vi "Setup Statically-Linked subWorkers.vi"(8 "error in":errorcluster, 11 "UI SmarAct in":refnum<class "UI SmarAct.lvclass">) -> (0 "error out":errorcluster, 3 "UI SmarAct out":refnum<class "UI SmarAct.lvclass">)   [LabVIEW 2024, in "UI SmarAct.lvclass"]
doc: "This VI performs a setup of all the statically-linked subWorkers that belong to the Worker that owns this VI. This VI must be called <b>before</b> any statically-linked subWorkers are called."
uses:
  UI SmarAct.lvclass
  UI SmarAct.lvclass/UI SmarAct.ctl
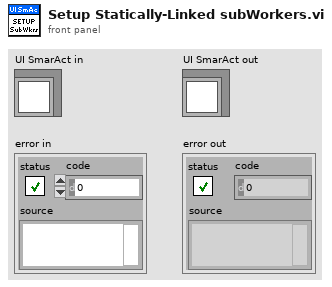
[diagram p1: front panel]
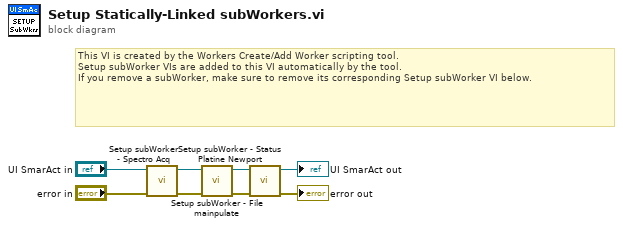
[diagram p0: block diagram]
diagram:
  # "This VI is created by the Workers Create/Add Worker scripting tool.\nSetup subWorker VIs are added to this VI automatically by the tool.\nIf you remove a subWorker, make sure to remove its corresponding Setup subWorker VI below."
  n1 = call "Setup subWorker - Spectro Acq.vi"("error in"="error in", "UI SmarAct in"="UI SmarAct in") -> ("error out"=w7:errorcluster, "UI SmarAct out"=w4:refnum<class "UI SmarAct.lvclass">)  [unwired: 8 in]
  n2 = call "Setup subWorker - File mainpulate.vi"("error in"=w7, "UI SmarAct in"=w4) -> ("error out"=w5:errorcluster, "UI SmarAct out"=w2:refnum<class "UI SmarAct.lvclass">)  [unwired: 8 in]
  n3 = call "Setup subWorker - Status Platine Newport.vi"("error in"=w5, "UI SmarAct in"=w2) -> ("error out"=→"error out":errorcluster, "UI SmarAct out"=→"UI SmarAct out":refnum<class "UI SmarAct.lvclass">)  [unwired: 8 in]
